vi "Copy File to Data Directory.vi"(8 "error in (no error)":errorcluster, 10 "Target File Directory":path, 11 "Installation Path":path) -> (0 "error out":errorcluster)   [LabVIEW 2019, in "NIPKG Packager.lvclass"]
doc: "Copies a file from the Installation Path to the Target File Directory. This is primarily intended for use with lvlibp paths."
uses:
  NIPKG Packager.lvclass
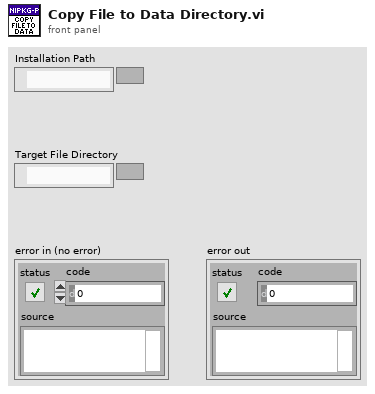
[diagram p1: front panel]
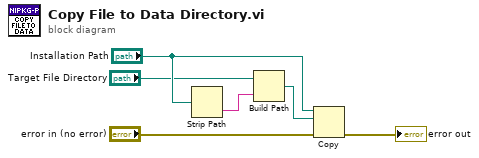
[diagram p0: block diagram]
diagram:
  n1 = Strip Path(path="Installation Path") -> (name=w3:string)  [unwired: 1 out]
  n2 = Build Path(base path="Target File Directory", name or relative path=w3) -> (appended path=w4:path)
  n3 = Copy(8:"error in (no error)", 10:w4, 11:"Installation Path") -> (0:→"error out":errorcluster)  [unwired: 2 in, 2 out]
